vi "UIRefs State.vi"(8 "error in (no error)":errorcluster, 11 "Mech Pump in":refnum<class "Mech Pump.lvclass">) -> (0 "error out":errorcluster, 3 "Mech Pump out":refnum<class "Mech Pump.lvclass">)   [LabVIEW 2021, in "Mech Pump.lvlib" / "Mech Pump.lvclass"]
uses:
  Mech Pump.lvclass
  Mech Pump.lvclass/Mech Pump.ctl
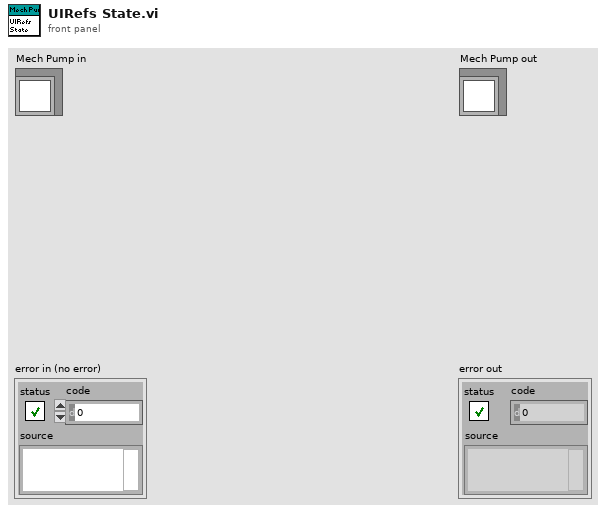
[diagram p1: front panel]
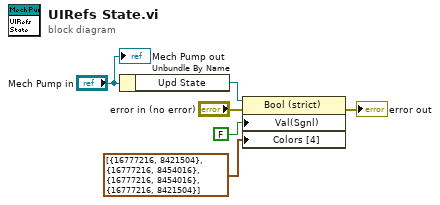
[diagram p0: block diagram]
diagram:
  n1 = Unbundle By Name("Mech Pump in") -> ("Upd State"=w6:refnum<vi>)
  n2 = property class="Bool (strict)"(reference=w6, error in="error in (no error)", "Val(Sgnl)"=FALSE ("Value (Signaling)"), "Colors [4]"=cluster{u32, u32}[] [{16777216, 8421504}, {16777216, 8454016}, {16777216, 8454016}, {16777216, 8421504}]) -> (error out=→"error out":errorcluster)  [unwired: 1 out]
  "Mech Pump out" <- "Mech Pump in"
